vi "to_xml.vi"(8 "error in":errorcluster, 11 "DDS Settings":T1={"Enable DDS"=TRUE, "Array of DDS Boxes"=[{"DDS box device reference"={"NI USB-8451 device reference"="USB0::0x3923::0x7166::01574F57::RAW", "DIO port"=0, "Serial Clock Rate [kHz]"=1000}, "Array of DDS Channels (4)"=[{"Power"=FALSE, "Channel Parameters"={"Ref Clock Rate [kHz]"=1000.0, "Full Scale Output\nPower [dBm]"=0.0}, "RAM Enable"=FALSE, "RAM Dest Type"=0, "RAM Default"={"Frequency [MHz]"=0.0, "Amplitude [dBm]"=0.0, "Phase Offset [rad]"=0.0}, "Array of DDS Profiles (8)"=[], "description"=""}, {"Power"=FALSE, "Channel Parameters"={"Ref Clock Rate [kHz]"=1000.0, "Full Scale Output\nPower [dBm]"=0.0}, "RAM Enable"=FALSE, "RAM Dest Type"=0, "RAM Default"={"Frequency [MHz]"=0.0, "Amplitude [dBm]"=0.0, "Phase Offset [rad]"=0.0}, "Array of DDS Profiles (8)"=[], "description"=""}, {"Power"=FALSE, "Channel Parameters"={"Ref Clock Rate [kHz]"=1000.0, "Full Scale Output\nPower [dBm]"=0.0}, "RAM Enable"=FALSE, "RAM Dest Type"=0, "RAM Default"={"Frequency [MHz]"=0.0, "Amplitude [dBm]"=0.0, "Phase Offset [rad]"=0.0}, "Array of DDS Profiles (8)"=[], "description"=""}, {"Power"=FALSE, "Channel Parameters"={"Ref Clock Rate [kHz]"=1000.0, "Full Scale Output\nPower [dBm]"=0.0}, "RAM Enable"=FALSE, "RAM Dest Type"=0, "RAM Default"={"Frequency [MHz]"=0.0, "Amplitude [dBm]"=0.0, "Phase Offset [rad]"=0.0}, "Array of DDS Profiles (8)"=[], "description"=""}], "Enable"=TRUE, "description"=""}, {"DDS box device reference"={"NI USB-8451 device reference"="USB0::0x3923::0x7166::01574FA5::RAW", "DIO port"=0, "Serial Clock Rate [kHz]"=1000}, "Array of DDS Channels (4)"=[{"Power"=FALSE, "Channel Parameters"={"Ref Clock Rate [kHz]"=1000.0, "Full Scale Output\nPower [dBm]"=0.0}, "RAM Enable"=FALSE, "RAM Dest Type"=0, "RAM Default"={"Frequency [MHz]"=0.0, "Amplitude [dBm]"=0.0, "Phase Offset [rad]"=0.0}, "Array of DDS Profiles (8)"=[], "description"=""}, {"Power"=FALSE, "Channel Parameters"={"Ref Clock Rate [kHz]"=1000.0, "Full Scale Output\nPower [dBm]"=0.0}, "RAM Enable"=FALSE, "RAM Dest Type"=0, "RAM Default"={"Frequency [MHz]"=0.0, "Amplitude [dBm]"=0.0, "Phase Offset [rad]"=0.0}, "Array of DDS Profiles (8)"=[], "description"=""}, {"Power"=FALSE, "Channel Parameters"={"Ref Clock Rate [kHz]"=1000.0, "Full Scale Output\nPower [dBm]"=0.0}, "RAM Enable"=FALSE, "RAM Dest Type"=0, "RAM Default"={"Frequency [MHz]"=0.0, "Amplitude [dBm]"=0.0, "Phase Offset [rad]"=0.0}, "Array of DDS Profiles (8)"=[], "description"=""}, {"Power"=FALSE, "Channel Parameters"={"Ref Clock Rate [kHz]"=1000.0, "Full Scale Output\nPower [dBm]"=0.0}, "RAM Enable"=FALSE, "RAM Dest Type"=0, "RAM Default"={"Frequency [MHz]"=0.0, "Amplitude [dBm]"=0.0, "Phase Offset [rad]"=0.0}, "Array of DDS Profiles (8)"=[], "description"=""}], "Enable"=TRUE, "description"=""}]} {"Array of DDS Boxes"."Array of DDS Channels (4)"."Channel Parameters"."Ref Clock Rate [kHz]" min=0.0}) -> (0 "error out":errorcluster, 3 "DDS settings string":string)   [LabVIEW 2013]
doc: "Creates xml from a DDS settings cluster in the format:\n\n<EnableDDS>%b</EnableDDS>\n<ArrayOfDDSBoxes>\n\n<box>\n<Enable>%b</Enable>\n<DDSBoxDeviceReference.Resource>%s</DDSBoxDeviceReference.Resource>\n<DDSBoxDeviceReference.DIOPort>%u</DDSBoxDeviceReference.DIOPort>\n<DDSBoxDeviceReference.SerialClockRate units=\"kHz\">%u</DDSBoxDeviceReference.SerialClockRate>\n<ArrayOfDDSChannels>\n\n<channel>\n<Power>%b</Power>\n<ChannelParameters.RefClockRate units=\"kHz\">%f</ChannelParameters.RefClockRate>\n<ChannelParameters.FullScaleOutputPower units=\"dBm\">%f</ChannelParameters.FullScaleOutputPower>\n<RAMEnable>%b</RAMEnable>\n<RAMDestType>%u</RAMDestType>\n<RAMDefault.Frequency units=\"MHz\">%s</RAMDefault.Frequency>\n<RAMDefault.Amplitude units=\"dBm\">%s</RAMDefault.Amplitude>\n<RAMDefault.Phase units=\"rad\">%s</RAMDefault.Phase>\n<ArrayOfDDSProfiles>\n\n<profile>\n<SingleTone.Frequency units=\"MHz\">%s</SingleTone.Frequency>\n<SingleTone.Amplitude units=\"dBm\">%s</SingleTone.Amplitude>\n<SingleTone.Phase units=\"rad\">%s</SingleTone.Phase>\n<RAMMode>%u</RAMMode>\n<ZeroCrossing>%b</ZeroCrossing>\n<NoDwellHigh>%b</NoDwellHigh>\n<FunctionOrStatic>%b</FunctionOrStatic>\n<RAMFunctionSettings>%s</RAMFunctionSettings>\n<RAMStaticArray>%s</RAMStaticArray>\n</profile>\n\n</ArrayOfDDSProfiles>\n</channel>\n\n</ArrayOfDDSChannels>\n</box>\n\n</ArrayOfDDSBoxes>\n\nMTL 2012 Dec 31"
uses:
  DDS drivers v3/DDS RAM mode.ctl
  <vilib>/ni845x/ni845x.llb/ni845xControl.ctl
  DDS drivers v3/DDS_box_device_reference.ctl
  DDS drivers v3/DDS_box_cluster.ctl
  DDS drivers v3/Array_of_DDS_Boxes.ctl
  DDS_Settings_Cluster.ctl
  DDS drivers v3/DDS_profile.ctl
  DDS drivers v3/DDS_channel.ctl
  DDS.lvclass
  DDS drivers v3/array_of_DDS_profiles.ctl
  DDS drivers v3/array_of_DDS_channels.ctl
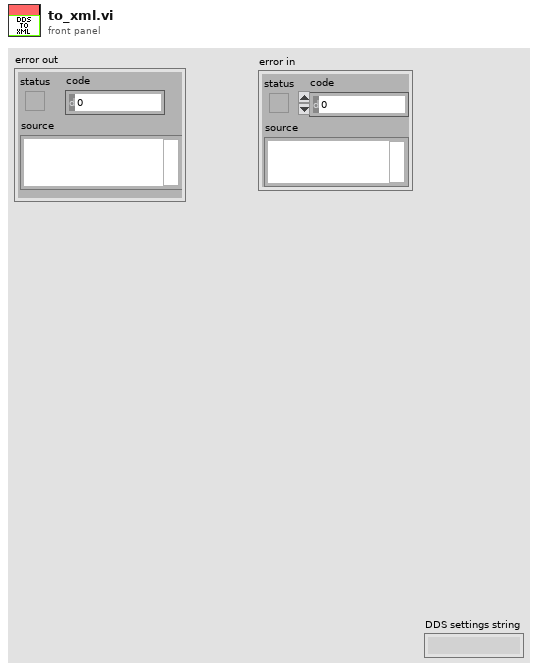
[diagram p1: front panel]
types:
  T1 = typedef "DDS_Settings_Cluster.ctl" = cluster{"Enable DDS":bool, "Array of DDS Boxes":T2}
  T2 = typedef "Array_of_DDS_Boxes.ctl" = T3[]
  T3 = typedef "DDS_box_cluster.ctl" = cluster{"DDS box device reference":T4, "Array of DDS Channels (4)":T6, "Enable":bool, "description":string}
  T4 = typedef "DDS_box_device_reference.ctl" = cluster{"NI USB-8451 device reference":T5, "DIO port":u8, "Serial Clock Rate [kHz]":u16}
  T5 = typedef "ni845xControl.ctl" = refnum<k21>
  T6 = typedef "DDS.lvclass/array_of_DDS_channels.ctl" = T7[]
  T7 = typedef "DDS.lvclass/DDS_channel.ctl" = cluster{"Power":bool, "Channel Parameters":cluster{"Ref Clock Rate [kHz]":dbl, "Full Scale Output\nPower [dBm]":dbl}, "RAM Enable":bool, "RAM Dest Type":u8, "RAM Default":cluster{"Frequency [MHz]":dbl, "Amplitude [dBm]":dbl, "Phase Offset [rad]":dbl}, "Array of DDS Profiles (8)":T8, "description":string}
  T8 = typedef "DDS.lvclass/array_of_DDS_profiles.ctl" = T9[]
  T9 = typedef "DDS_profile.ctl" = cluster{"Single Tone":cluster{"Frequency [MHz]":dbl, "Amplitude [dBm]":dbl, "Phase Offset [rad]":dbl}, "RAM Mode ":T10, "Zero-crossing":bool, "No Dwell High":bool, "Function/Static":bool, "RAM Function Settings":string[], "RAM Static Array":dbl[], "description":string}
  T10 = typedef "DDS RAM mode.ctl" = enum16{"Direct Switch", "Ramp Up", "Bidirectional Ramp", "Continuous Bidirectional Ramp", "Continuous Recirculate", "Direct Switch 2", "Direct Switch 3", "Direct Switch 4"}
  T11 = cluster{"Ref Clock Rate [kHz]":dbl, "Full Scale Output\nPower [dBm]":dbl}
  T12 = cluster{"Frequency [MHz]":dbl, "Amplitude [dBm]":dbl, "Phase Offset [rad]":dbl}
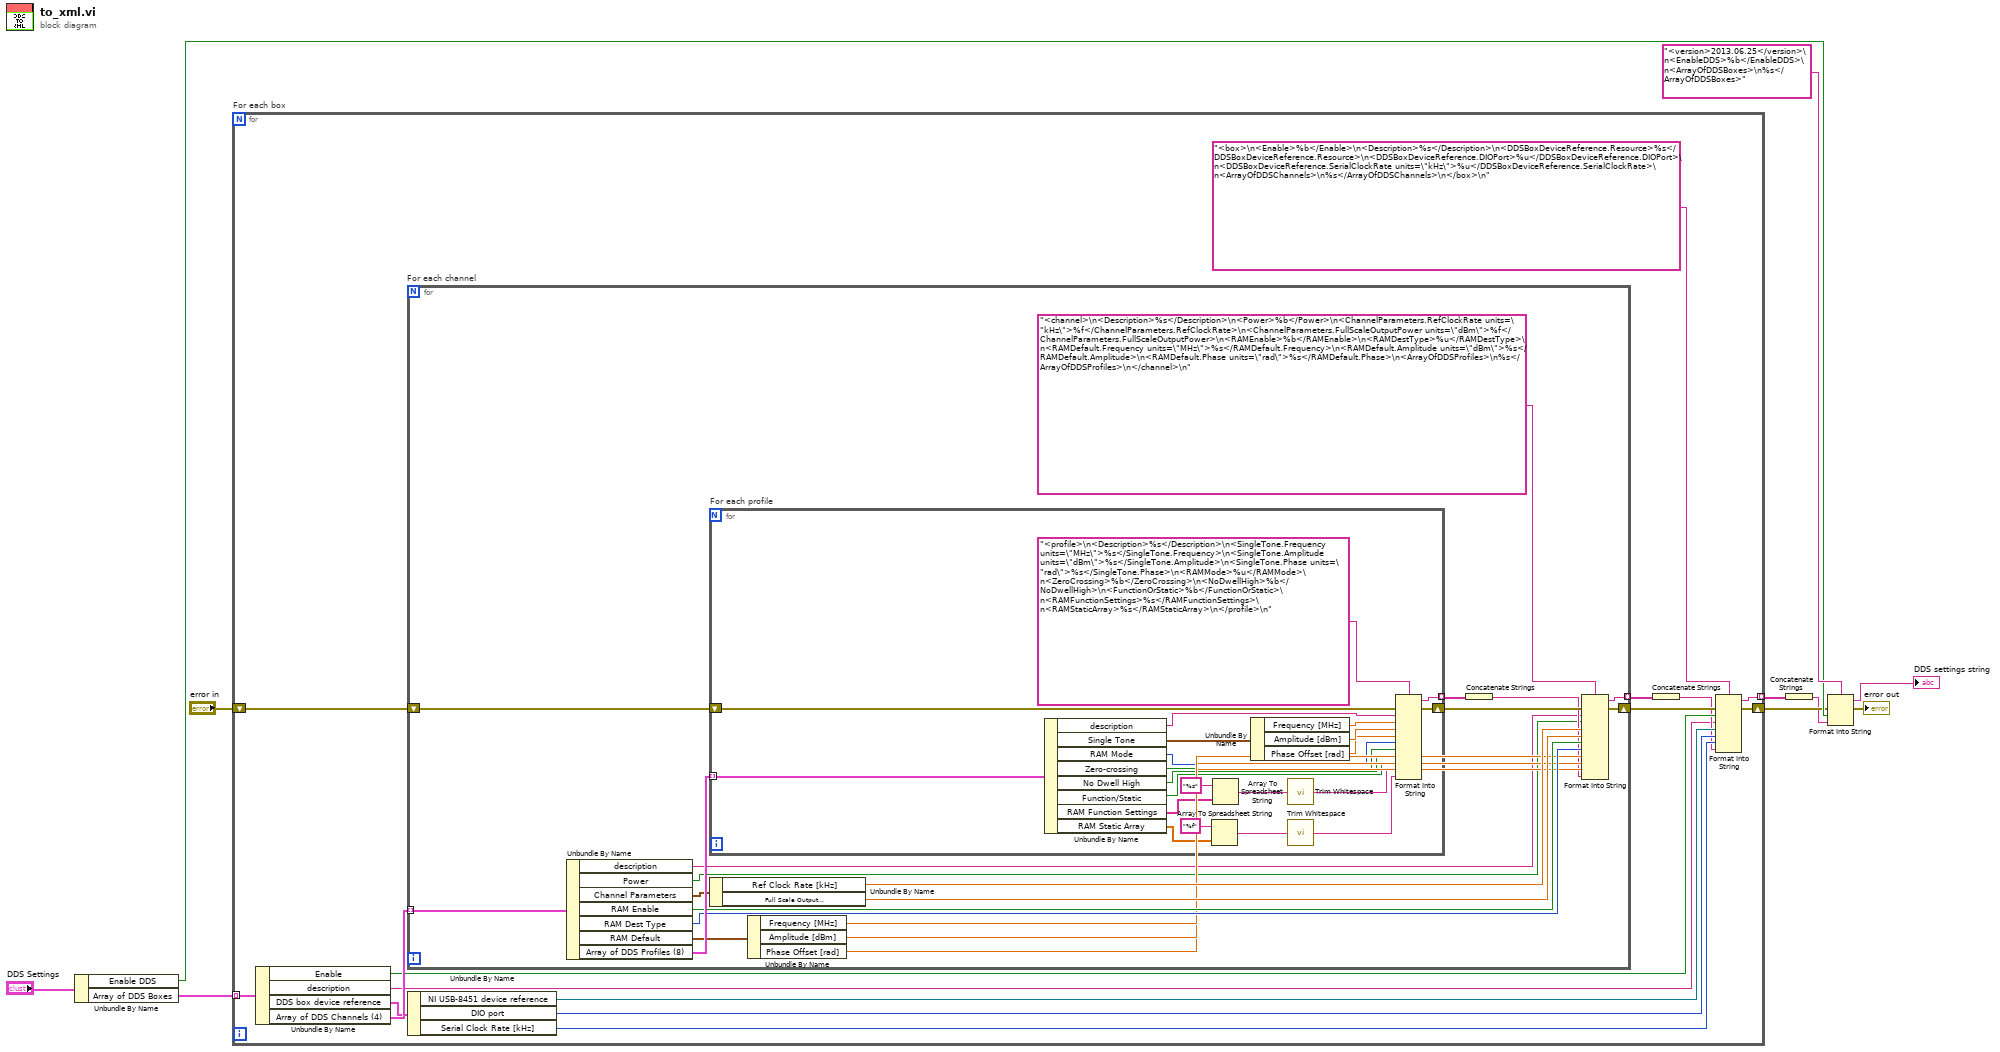
[diagram p0: block diagram]
diagram:
  n1 = Unbundle By Name("DDS Settings") -> ("Enable DDS"=w6:bool, "Array of DDS Boxes"=w5:T2)
  n2 = for "For each box" {
    tunnel: w5 -> [w25] mode=indexing
    shift-right: [w16] -> w3
    shift-left: "error in" -> [w18]
    tunnel: [w14] -> w2 mode=indexing
    n3 = Unbundle By Name(w25) -> ("Enable"=w15:bool, "description"=w11:string, "DDS box device reference"=w23:T4, "Array of DDS Channels (4)"=w24:T6)
    n4 = for "For each channel" {
      tunnel: w24 -> [w45] mode=indexing
      shift-right: [w38] -> w17
      shift-left: w18 -> [w40]
      tunnel: [w41] -> w13 mode=indexing
      n5 = Unbundle By Name(w45) -> ("description"=w27:string, "Power"=w26:bool, "Channel Parameters"=w43:T11, "RAM Enable"=w34:bool, "RAM Dest Type"=w33:u8, "RAM Default"=w42:T12, "Array of DDS Profiles (8)"=w44:T8)
      n6 = for "For each profile" {
        tunnel: w44 -> [w67] mode=indexing
        shift-right: [w63] -> w39
        shift-left: w40 -> [w62]
        tunnel: [w65] -> w29 mode=indexing
        n7 = Unbundle By Name(w67) -> ("description"=w47:string, "Single Tone"=w66:T12, "RAM Mode"=w49:T10, "Zero-crossing"=w50:bool, "No Dwell High"=w59:bool, "Function/Static"=w58:bool, "RAM Function Settings"=w57:string[], "RAM Static Array"=w56:dbl[])
        n8 = Array To Spreadsheet String(array=w56, 3:"%f" ("format string")) -> (spreadsheet string=w53:string)  [unwired: 1 in]
        n9 = Array To Spreadsheet String(array=w57, 3:"%s" ("format string")) -> (spreadsheet string=w48:string)  [unwired: 1 in]
        n10 = Unbundle By Name(w66) -> ("Frequency [MHz]"=w46:dbl, "Amplitude [dBm]"=w61:dbl, "Phase Offset [rad]"=w60:dbl)
        n11 = call <vilib>:"Trim Whitespace.vi"("string"=w48) -> ("trimmed string"=w54:string)  [unwired: 1 in]
        n12 = call <vilib>:"Trim Whitespace.vi"("string"=w53) -> ("trimmed string"=w52:string)  [unwired: 1 in]
        n13 = Format Into String(format string="<profile>\n<Description>%s</Description>\n<SingleTone.Frequency units=\"MHz\">%s</SingleTone.Frequency>\n<SingleTone.Amplitude units=\"dBm\">%s</SingleTone.Amplitude>\n<SingleTone.Phase units=\"rad\">%s</SingleTone.Phase>\n<RAMMode>%u</RAMMode>\n<ZeroCrossing>%b</ZeroCrossing>\n<NoDwellHigh>%b</NoDwellHigh>\n<FunctionOrStatic>%b</FunctionOrStatic>\n<RAMFunctionSettings>%s</RAMFunctionSettings>\n<RAMStaticArray>%s</RAMStaticArray>\n</profile>\n", error in=w62, w47, w46, w61, w60, w49, w50, w59, w58, w54, w52) -> (resulting string=w65:string, error out=w63:errorcluster)  [unwired: 1 in]
      }
      n14 = Unbundle By Name(w43) -> ("Ref Clock Rate [kHz]"=w36:dbl, "Full Scale Output\nPower [dBm]"=w35:dbl)
      n15 = Unbundle By Name(w42) -> ("Frequency [MHz]"=w32:dbl, "Amplitude [dBm]"=w31:dbl, "Phase Offset [rad]"=w30:dbl)
      n16 = Concatenate Strings(w29) -> (w28:string)
      n17 = Format Into String(format string="<channel>\n<Description>%s</Description>\n<Power>%b</Power>\n<ChannelParameters.RefClockRate units=\"kHz\">%f</ChannelParameters.RefClockRate>\n<ChannelParameters.FullScaleOutputPower units=\"dBm\">%f</ChannelParameters.FullScaleOutputPower>\n<RAMEnable>%b</RAMEnable>\n<RAMDestType>%u</RAMDestType>\n<RAMDefault.Frequency units=\"MHz\">%s</RAMDefault.Frequency>\n<RAMDefault.Amplitude units=\"dBm\">%s</RAMDefault.Amplitude>\n<RAMDefault.Phase units=\"rad\">%s</RAMDefault.Phase>\n<ArrayOfDDSProfiles>\n%s</ArrayOfDDSProfiles>\n</channel>\n", error in=w39, w27, w26, w36, w35, w34, w33, w32, w31, w30, w28) -> (resulting string=w41:string, error out=w38:errorcluster)  [unwired: 1 in]
    }
    n18 = Unbundle By Name(w23) -> ("NI USB-8451 device reference"=w21:T5, "DIO port"=w20:u8, "Serial Clock Rate [kHz]"=w19:u16)
    n19 = Concatenate Strings(w13) -> (w12:string)
    n20 = Format Into String(format string="<box>\n<Enable>%b</Enable>\n<Description>%s</Description>\n<DDSBoxDeviceReference.Resource>%s</DDSBoxDeviceReference.Resource>\n<DDSBoxDeviceReference.DIOPort>%u</DDSBoxDeviceReference.DIOPort>\n<DDSBoxDeviceReference.SerialClockRate units=\"kHz\">%u</DDSBoxDeviceReference.SerialClockRate>\n<ArrayOfDDSChannels>\n%s</ArrayOfDDSChannels>\n</box>\n", error in=w17, w15, w11, w21, w20, w19, w12) -> (resulting string=w14:string, error out=w16:errorcluster)  [unwired: 1 in]
  }
  n21 = Concatenate Strings(w2) -> (w1:string)
  n22 = Format Into String(format string="<version>2013.06.25</version>\n<EnableDDS>%b</EnableDDS>\n<ArrayOfDDSBoxes>\n%s</ArrayOfDDSBoxes>", error in=w3, w6, w1) -> (resulting string=→"DDS settings string":string, error out=→"error out":errorcluster)  [unwired: 1 in]
